vi "Photodode_read.vi"(6 "Error In":errorcluster, 8 "Sampling Time":dbl) -> (0 "error out":errorcluster, 2 "data":waveform(dbl)[](array[waveform]))   [LabVIEW 2017]
uses:
  <vilib>/DAQmx/read.llb/DAQmx Read (Analog 1D Wfm NChan NSamp).vi
  <vilib>/DAQmx/create/channels.llb/DAQmx Create Channel (AI-Voltage-Basic).vi
  <vilib>/DAQmx/configure/timing.llb/DAQmx Timing (Sample Clock).vi
  <vilib>/DAQmx/miscellaneous.llb/DAQmx Fill In Error Info.vi
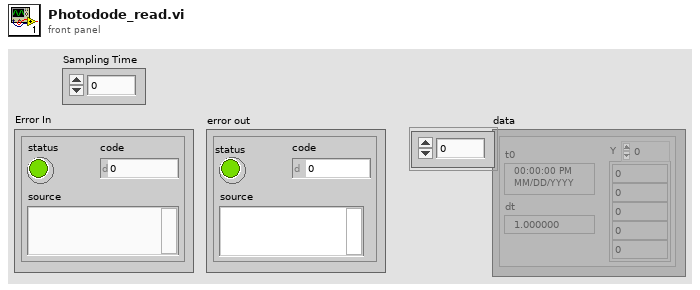
[diagram p1: front panel]
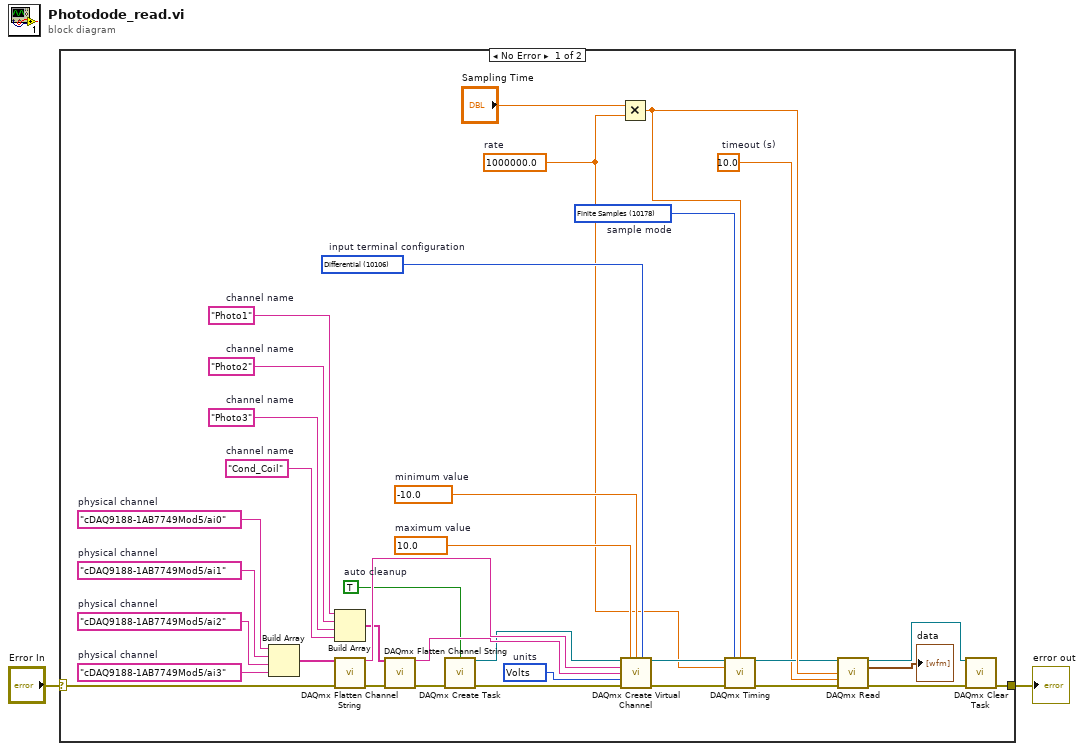
[diagram p0: block diagram]
diagram:
  n1 = case shown="No Error" "Error In" {
    selector: "Error In" -> [w4 w38]
    tunnel: [w5 w38] -> w2
    frame No Error {
      w13 = 10178 items=["Finite Samples"=10178, "Continuous Samples"=10123, "Hardware Timed Single Point"=12522]  # sample mode
      w16 = 1000000.0  # rate
      w25 = "Cond_Coil"  # channel name
      w33 = "cDAQ9188-1AB7749Mod5/ai3"  # physical channel
      w24 = "Photo3"  # channel name
      w30 = "cDAQ9188-1AB7749Mod5/ai2"  # physical channel
      w23 = "Photo2"  # channel name
      w29 = "cDAQ9188-1AB7749Mod5/ai1"  # physical channel
      w18 = 10106 items=["default"=-1, "RSE"=10083, "NRSE"=10078, "Differential"=10106, "Pseudodifferential"=12529]  # input terminal configuration
      w21 = 10348 items=["Volts"=10348, "From Custom Scale"=10065]  # units
      w22 = "Photo1"  # channel name
      w19 = -10.0  # minimum value
      w20 = 10.0  # maximum value
      w31 = "cDAQ9188-1AB7749Mod5/ai0"  # physical channel
      w11 = TRUE  # auto cleanup
      w7 = 10.0  # timeout (s)
      n2 = Build Array(w31, w29, w30, w33) -> (w28:string[])
      n3 = Build Array(w22, w23, w24, w25) -> (w26:string[])
      n4 = call <vilib>:"DAQmx Flatten Channel String.vi"("names in"=w28, "error in"=w4) -> ("names out"=w32:string, "error out"=w37:errorcluster)  [unwired: 12 in]
      n5 = call <vilib>:"DAQmx Flatten Channel String.vi"("names in"=w26, "error in"=w37) -> ("names out"=w27:string, "error out"=w36:errorcluster)  [unwired: 12 in]
      n6 = call <vilib>:"DAQmx Create Task.vi"("auto cleanup"=w11, "error in"=w36) -> ("task out"=w12:refnum<k21>, "error out"=w10:errorcluster)  [unwired: 12 in]
      n7 = Multiply(x="Sampling Time", y=w16) -> (x*y=w17:dbl)
      n8 = call-poly <vilib>:"DAQmx Create Virtual Channel.vi"("task in"=w12, "maximum value"=w20, "minimum value"=w19, "input terminal configuration"=w18, "physical channels"=w32, "name to assign"=w27, "units"=w21, "error in"=w10) -> ("task out"=w34:refnum<k21>, "error out"=w35:errorcluster)  [unwired: 6 in]
      n9 = call-poly <vilib>:"DAQmx Timing.vi"("task/channels in"=w34, "sample mode"=w13, "samples per channel"=w17, "rate"=w16, "error in"=w35) -> ("task out"=w14:refnum<k21>, "error out"=w15:errorcluster)  [unwired: 9 in]
      n10 = call-poly <vilib>:"DAQmx Read.vi"("task/channels in"=w14, "number of samples per channel"=w17, "timeout"=w7, "error in"=w15) -> ("task out"=w9:refnum<k21>, "data"=→"data":waveform(dbl)[], "error out"=w8:errorcluster)  [unwired: 9 in]
      n11 = call <vilib>:"DAQmx Clear Task.vi"("task in"=w9, "error in"=w8) -> ("error out"=w5:errorcluster)  [unwired: 13 in]
    }
    frame Error {
    }
  }
  "error out" <- w2
